vi "ExportConfigurationToFile.vi"(8 "error in (no error)":errorcluster, 11 "Node Ptr":u64 format="%.0x") -> (0 "error out":errorcluster)   [LabVIEW 2019, in "Instrument Addon System Explorer.lvlib"]
uses:
  Instrument Addon System Explorer.lvlib
  APIs/Scripting API/Instrument Addon Scripting API.lvlib
panel:
  in  "Tag":string
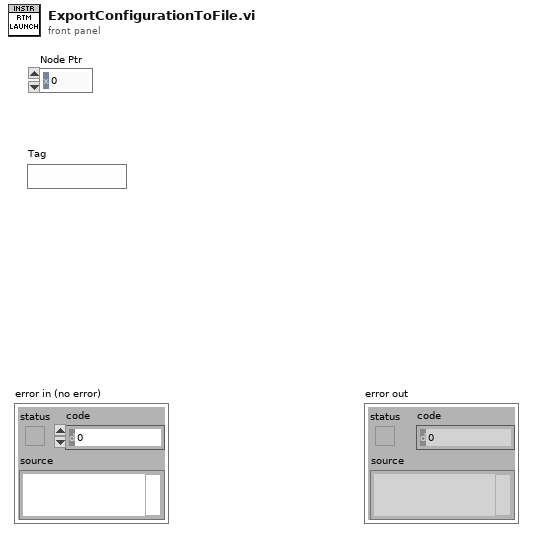
[diagram p1: front panel]
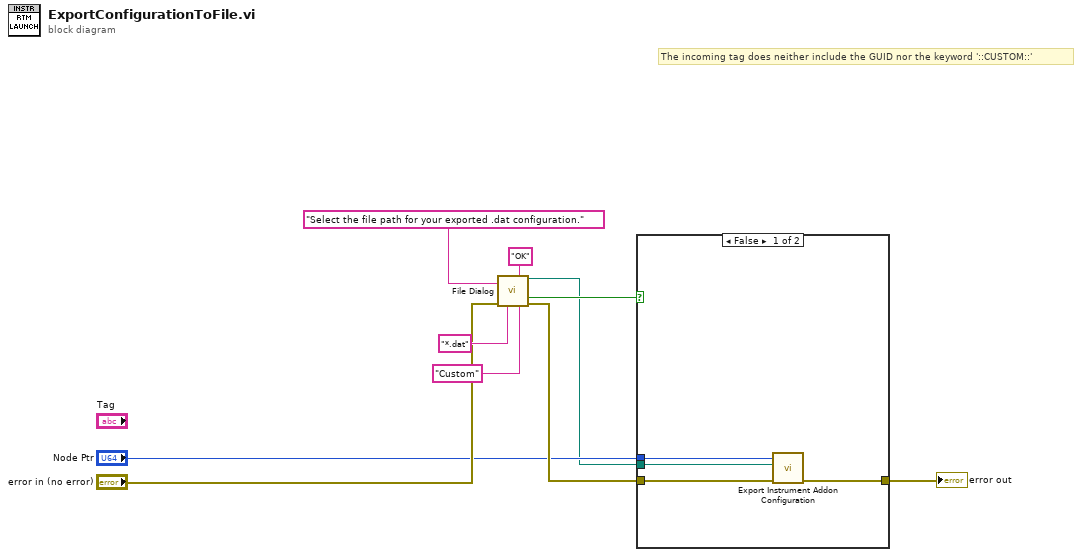
[diagram p0: block diagram]
diagram:
  # "The incoming tag does neither include the GUID nor the keyword '::CUSTOM::'"
  n1 = call "File Dialog"("prompt"="Select the file path for your exported .dat configuration.", "button label"="OK", "error in"="error in (no error)", "pattern (all files)"="*.dat" ("file extension"), "pattern label"="Custom") -> ("selected path"=w1:path, "cancelled"=w3:bool, "error out"=w4:errorcluster)  [unwired: 7 in, 1 out]
  n2 = case shown="False" w3 {
    tunnel: [w14 w15] -> w10
    tunnel: w4 -> [w13 w15]
    tunnel: "Node Ptr" -> [w12 _]
    tunnel: w1 -> [w11 _]
    frame False {
      n3 = call "Export Instrument Addon Configuration.vi"("error in (no error)"=w13, "export file path"=w11, "instrument addon refnum in"=w12) -> ("error out"=w14:errorcluster)  [unwired: 7 in, 1 out]
    }
    frame True {
    }
  }
  "error out" <- w10
